vi "topological_sort_(Kahn).vi"(8 "error in (no error)":errorcluster, 11 "DiGraph in":refnum<class "DiGraph.lvclass">) -> (0 "error out":errorcluster, 1 "cycle detected":bool, 2 "nodes (sorted)":refnum<class "Node.lvclass">[](array[class]))   [LabVIEW 2020, in "graph.lvlib" / "DiGraph.lvclass"]
uses:
  DiGraph.lvclass
  C:/Projects/labview-project-load-tools/source/submodules/graph-api-labview/source/api/Graph/Graph.lvclass
  Node/Node.lvclass
  DiGraph.lvclass/DiGraph.ctl
  Graph/Graph.lvclass/Graph.ctl
  ID/ID.lvclass
  Graph/Graph.lvclass
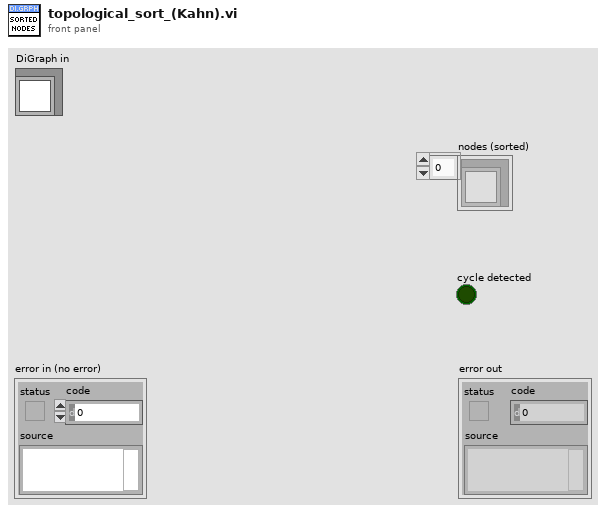
[diagram p1: front panel]
types:
  T1 = map{refnum<class "ID.lvclass">, set{refnum<class "ID.lvclass">}}
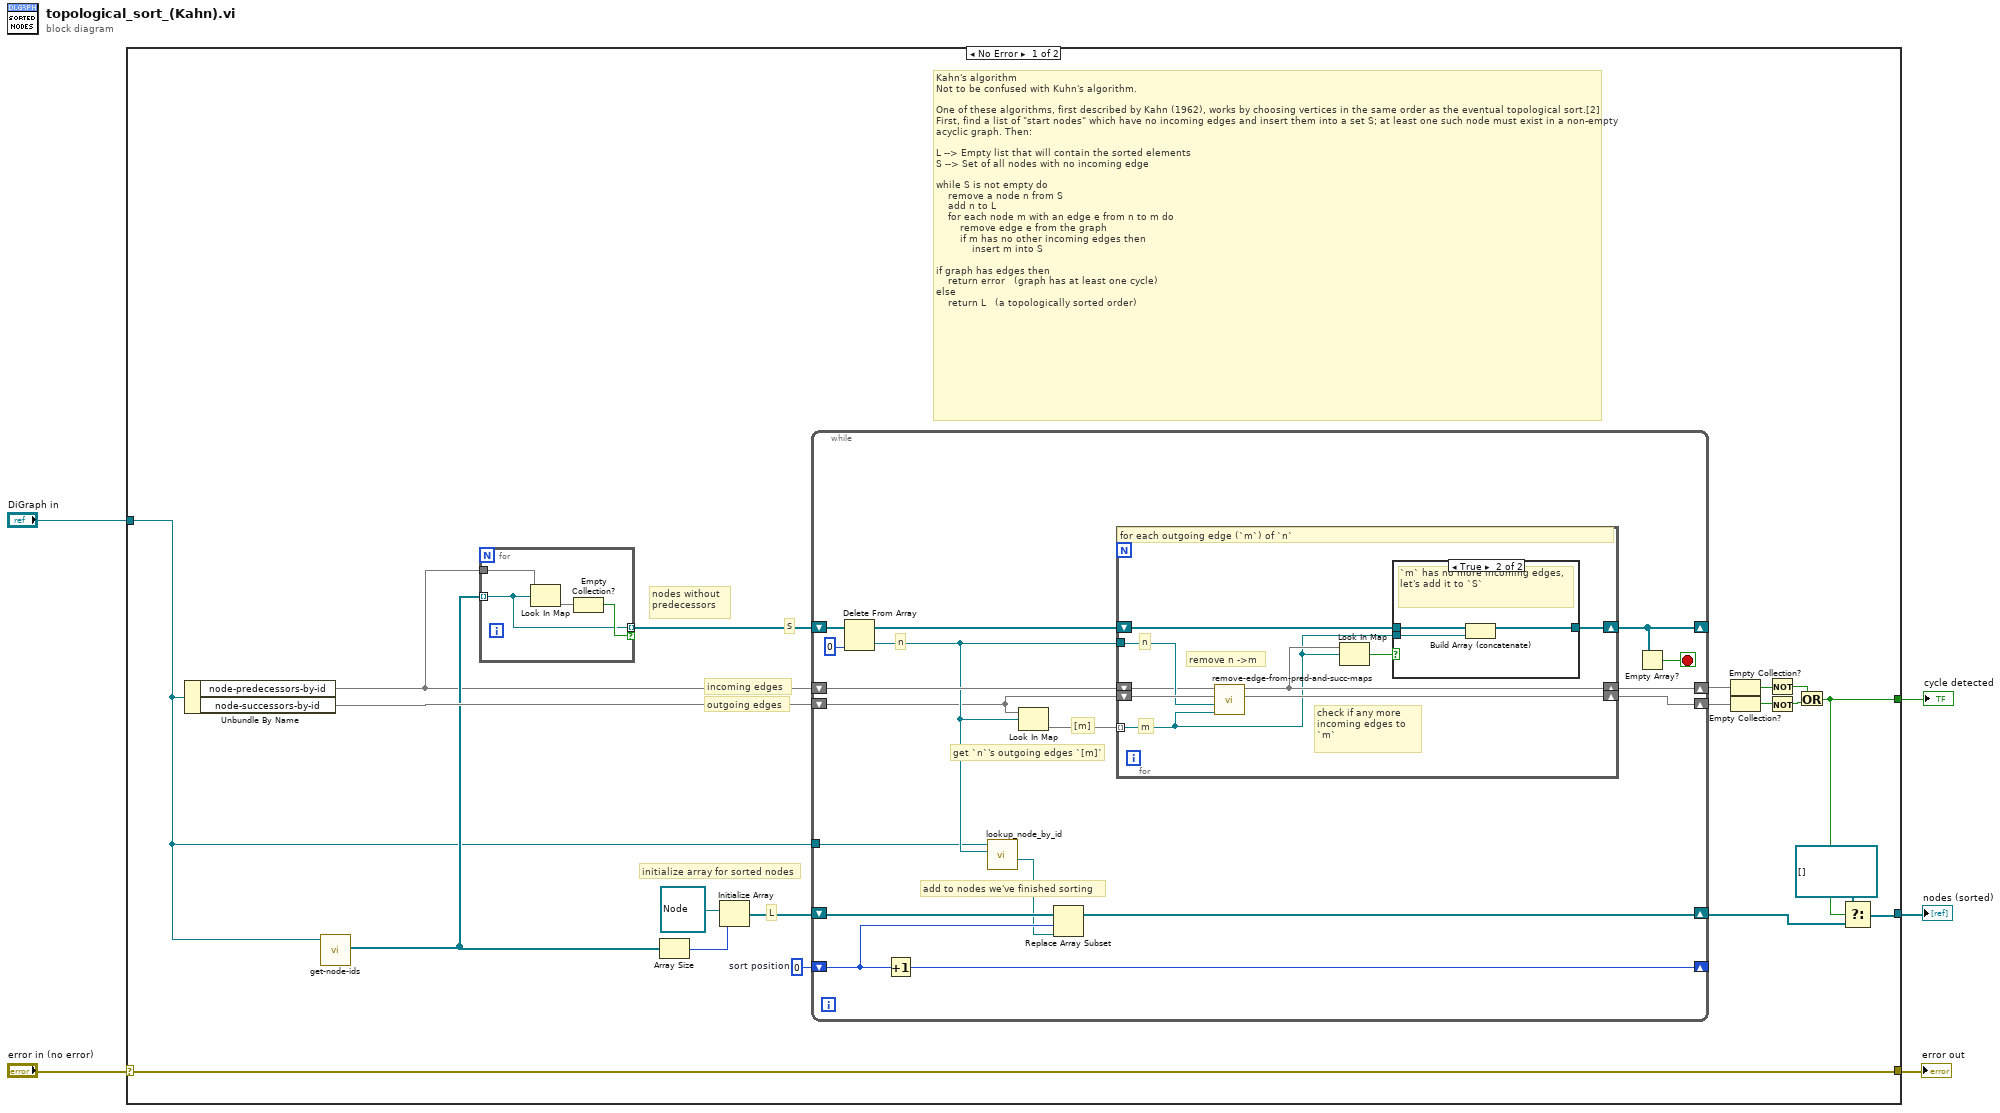
[diagram p0: block diagram]
diagram:
  n1 = case shown="No Error" "error in (no error)" {
    selector: "error in (no error)" -> [w6 w60]
    tunnel: [w6 w60] -> w4
    tunnel: "DiGraph in" -> [w7 _]
    tunnel: [w11 _] -> w2
    tunnel: [w9 _] -> w1
    frame No Error {
      w24 = 0  # sort position
      # "initialize array for sorted nodes"
      # "Kahn's algorithm\nNot to be confused with Kuhn's algorithm.\n\nOne of these algorithms, first described by Kahn (1962), works by choosing vertices in the same order as the eventual topological sort.[2] First, find a list of \"start nodes\" which have no incoming edges and insert them into a set S; at least one such node must exist in a non-empty acyclic graph. Then:\n\nL --> Empty list that will contain the sorted elements\nS --> Set of all nodes with no incoming edge\n\nwhile S is not empty do\n    remove a node n from S\n    add n to L\n    for each node m with an edge e from n to m do\n        remove edge e from the graph\n        if m has no other incoming edges then\n            insert m into S\n\nif graph has edges then\n    return error   (graph has at least one cycle)\nelse \n    return L   (a topologically sorted order)"
      # "outgoing edges"
      # "incoming edges"
      # "L"
      # "S"
      # "nodes without predecessors"
      n2 = Unbundle By Name(w7) -> ("node-predecessors-by-id"=w12:T1, "node-successors-by-id"=w23:T1)
      n3 = call "get-node-ids.vi"("Graph in"=w7) -> ("node-ids"=w13:refnum<class "ID.lvclass">[])  [unwired: 10 in]
      n4 = for {
        tunnel: w13 -> [w56] mode=indexing
        tunnel: w12 -> [w59]
        tunnel: [w56] -> w25 mode=indexing if=w58
        n5 = Look In Map(map=w59, key=w56) -> (value=w57:set{refnum<class "ID.lvclass">})  [unwired: 1 in, 1 out]
        n6 = Empty Collection?(1:w57) -> (0:w58:bool)
      }
      n7 = Array Size(array=w13) -> (size(s)=w14:i32)
      n8 = Initialize Array(refnum<class "Node.lvclass"> refnum ("node"), w14) -> (w16:refnum<class "Node.lvclass">[])
      n9 = while {
        shift-right: [w38] -> w10
        shift-left: w16 -> [w41]
        shift-right: [w31] -> _
        shift-left: w25 -> [w42]
        shift-right: [w39] -> _
        shift-left: w24 -> [w40]
        shift-right: [w37] -> w22
        shift-left: w12 -> [w34]
        shift-right: [w36] -> w21
        shift-left: w23 -> [w27]
        tunnel: w7 -> [w28]
        stop <- w30 stop-if-true
        # "add to nodes we've finished sorting"
        # "[m]"
        # "get `n`'s outgoing edges `[m]`"
        # "n"
        n10 = Delete From Array(array=w42, index=0) -> (deleted portion=w29:refnum<class "ID.lvclass">, array with subset deleted=w33:refnum<class "ID.lvclass">[])  [unwired: 1 in]
        n11 = Increment(x=w40) -> (x+1=w39:i32)
        n12 = call "lookup_node_by_id.vi"("node_id"=w29, "graph"=w28) -> ("node"=w26:refnum<class "Node.lvclass">)  [unwired: 8 in, 1 out]
        n13 = Look In Map(map=w27, key=w29) -> (value=w35:set{refnum<class "ID.lvclass">})  [unwired: 1 in, 1 out]
        n14 = Replace Array Subset(array=w41, new element=w26, index=w40) -> (w38:refnum<class "Node.lvclass">[])
        n15 = for {
          tunnel: w29 -> [w49]
          shift-right: [w47] -> w37
          shift-left: w34 -> [w48]
          shift-right: [w50] -> w36
          shift-left: w27 -> [w51]
          tunnel: w35 -> [w44] mode=indexing
          shift-right: [w43] -> w31
          shift-left: w33 -> [w45]
          # "remove n ->m"
          # "n"
          # "check if any more incoming edges to `m`"
          # "m"
          # "for each outgoing edge (`m`) of `n`"
          n16 = call "remove-edge-from-pred-and-succ-maps.vi"("sink-id"=w44, "source-id"=w49, "node-successors-by-id"=w51, "node-predecessors-by-id"=w48) -> ("node-successors-by-id out"=w50:T1, "node-predecessors-by-id out"=w47:T1)  [unwired: 6 in]
          n17 = Look In Map(map=w47, key=w44) -> (key not found?=w46:bool)  [unwired: 1 in, 1 out]
          n18 = case shown="True" w46 {
            tunnel: w45 -> [w52 w55]
            tunnel: w44 -> [_ w54]
            tunnel: [w52 w53] -> w43
            frame False {
            }
            frame True {
              # "`m` has no more incoming edges, let's add it to `S`"
              n19 = Build Array (concatenate)(w55, w54) -> (w53:refnum<class "ID.lvclass">[])
            }
          }
        }
        n20 = Empty Array?(array=w31) -> (empty?=w30:bool)
      }
      n21 = Empty Collection?(1:w22) -> (0:w19:bool)
      n22 = Empty Collection?(1:w21) -> (0:w20:bool)
      n23 = Not(x=w19) -> (.not. x?=w18:bool)
      n24 = Not(x=w20) -> (.not. x?=w17:bool)
      n25 = Or(x=w18, y=w17) -> (x .or. y?=w11:bool)
      n26 = Select(t=refnum<class "Node.lvclass">[] [], s=w11, f=w10) -> (s? t:f=w9:refnum<class "Node.lvclass">[])
    }
    frame Error {
    }
  }
  "error out" <- w4
  "cycle detected" <- w2
  "nodes (sorted)" <- w1
